vi "Do Set Value.vi"(8 "error in (no error)":errorcluster, 10 "set_value Argument":T3, 11 "Data Cluster in":T1) -> (0 "error out":errorcluster, 3 "Data Cluster out":T1)   [LabVIEW 2025, in "Scripting Server.lvlib"]
uses:
  Scripting Server.lvlib
  Module Data--cluster.ctl
  Config Data.ctl
  set_value Argument--cluster.ctl
  set_value (Reply Payload)--cluster.ctl
  <vilib>/Utility/error.llb/Error Cluster From Error Code.vi
  <vilib>/ErrorRing/Error Ring.xnode
panel:
  out "Class Name":string
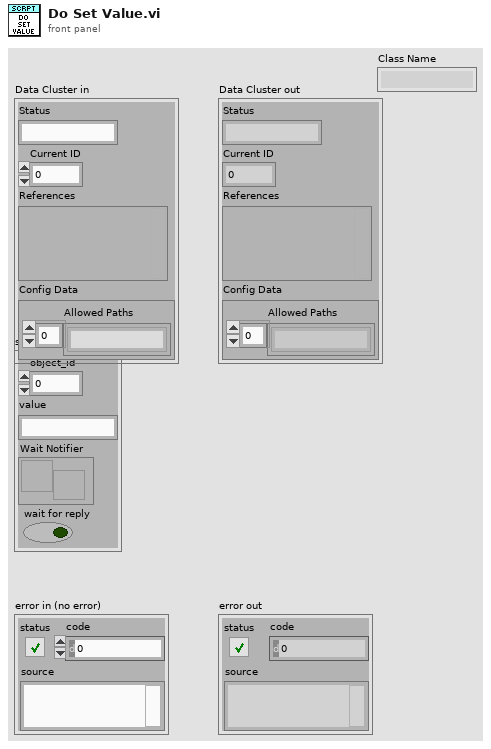
[diagram p1: front panel]
types:
  T1 = typedef "Scripting Server.lvlib/Module Data--cluster.ctl" = cluster{"Status":string, "Current ID":i32, "References":variant, "Config Data":T2}
  T2 = typedef "Scripting Server.lvlib/Config Data.ctl" = cluster{"Allowed Paths":string[]}
  T3 = typedef "Scripting Server.lvlib/set_value Argument--cluster.ctl" = cluster{"object_id":i32, "value":string, "Wait Notifier":refnum<notifier>, "wait for reply":bool}
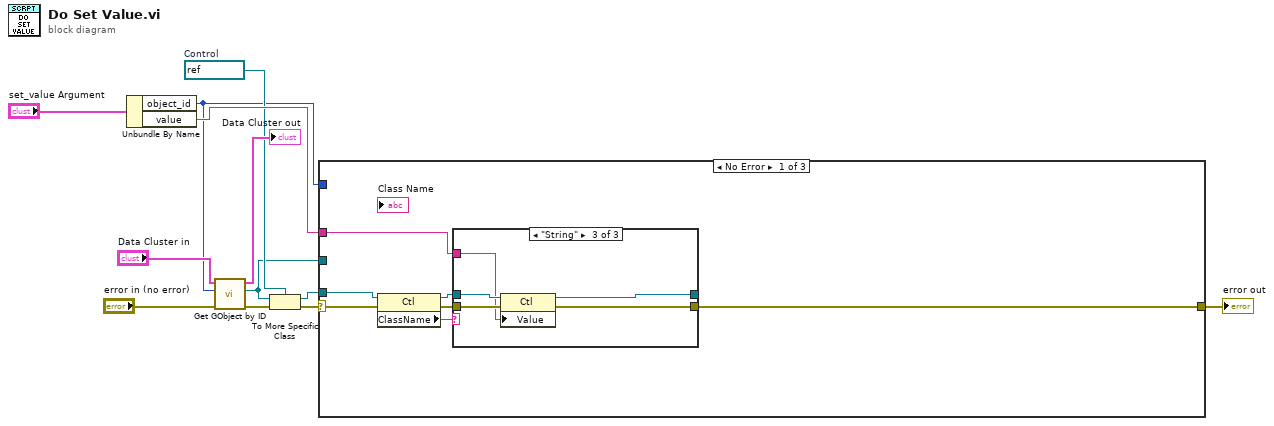
[diagram p0: block diagram]
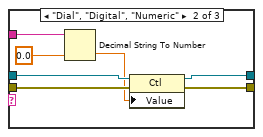
[diagram p3: hidden frame]
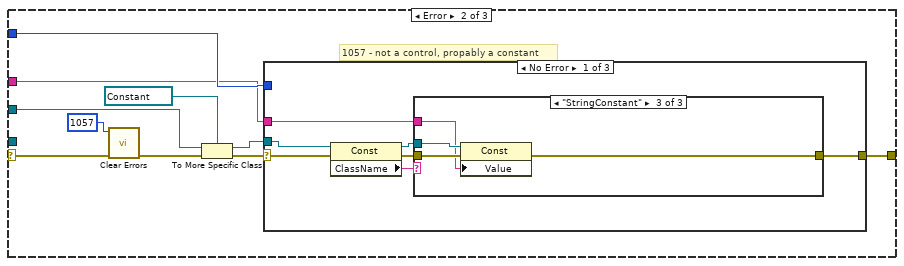
[diagram p4: hidden frame]
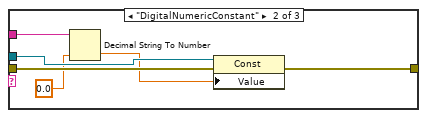
[diagram p6: hidden frame]
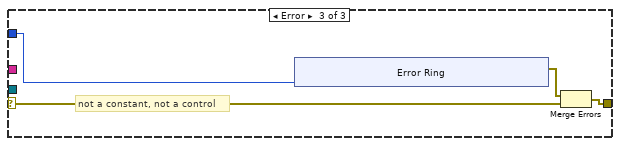
[diagram p8: hidden frame]
diagram:
  w6 = refnum<vi> refnum  # Control
  n1 = Unbundle By Name("set_value Argument") -> ("object_id"=w2:i32, "value"=w7:string)
  n2 = call "Get GObject by ID.vi"("error in (no error)"="error in (no error)", "ID"=w2, "Data Cluster in"="Data Cluster in") -> ("error out"=w4:errorcluster, "gobject"=w1:refnum<vi>, "Data Cluster out"=→"Data Cluster out":T1)  [unwired: 6 in]
  n3 = To More Specific Class(target class=w6, reference=w1, error in=w4) -> (specific class reference=w3:refnum<vi>, error out=w5:errorcluster)
  n4 = case shown="No Error" w5 {
    selector: w5 -> [w19 w43 w74]
    tunnel: w3 -> [w15 _ _]
    tunnel: [w18 w41 w74] -> w8
    tunnel: w7 -> [w17 w37 _]
    tunnel: w2 -> [_ w38 _]
    tunnel: w1 -> [_ w36 _]
    frame No Error {
      n5 = property class="Ctl"(reference=w15, error in=w19) -> (reference out=w14:refnum<vi>, error out=w16:errorcluster, "ClassName"=w13:string)
      n6 = case shown="\"String\"" w13 {
        tunnel: w16 -> [w20 w28 w33]
        tunnel: [w20 w27 w32] -> w18
        tunnel: w14 -> [w21 w26 w31]
        tunnel: [w21 w25 w30] -> _
        tunnel: w17 -> [_ w24 w29]
        frame "False", Default {
        }
        frame "Dial", "Digital", "Numeric" {
          n7 = Decimal String To Number(string=w24, default (0L)=0.0) -> (number=w23:dbl)  [unwired: 1 in, 1 out]
          n8 = property class="Ctl"(reference=w26, error in=w28, "Value"=w23) -> (reference out=w25:refnum<vi>, error out=w27:errorcluster)
        }
        frame "String" {
          n9 = property class="Ctl"(reference=w31, error in=w33, "Value"=w29) -> (reference out=w30:refnum<vi>, error out=w32:errorcluster)
        }
      }
    }
    frame Error {
      # "1057 - not a control, propably a constant"
      n10 = call <vilib>:"Clear Errors.vi"("error in (no error)"=w43, "specific error code to clear (0: all)"=1057) -> ("error out"=w35:errorcluster)  [unwired: 4 in, 1 out]
      n11 = To More Specific Class(target class=refnum<vi> refnum ("reference"), reference=w36, error in=w35) -> (specific class reference=w40:refnum<vi>, error out=w39:errorcluster)
      n12 = case shown="No Error" w39 {
        selector: w39 -> [w48 w62 w66]
        tunnel: [w47 w62 w64] -> w41
        tunnel: w40 -> [w49 _ _]
        tunnel: w38 -> [_ _ w65]
        tunnel: w37 -> [w44 _ _]
        frame No Error {
          n13 = property class="Const"(reference=w49, error in=w48) -> (reference out=w46:refnum<vi>, error out=w50:errorcluster, "ClassName"=w45:string)
          n14 = case shown="\"StringConstant\"" w45 {
            tunnel: w50 -> [w51 w57 w61]
            tunnel: [w51 w56 w60] -> w47
            tunnel: w46 -> [_ w55 w59]
            tunnel: w44 -> [_ w54 w58]
            frame "False", Default {
            }
            frame "DigitalNumericConstant" {
              n15 = Decimal String To Number(string=w54, default (0L)=0.0) -> (number=w53:dbl)  [unwired: 1 in, 1 out]
              n16 = property class="Const"(reference=w55, error in=w57, "Value"=w53) -> (error out=w56:errorcluster)  [unwired: 1 out]
            }
            frame "StringConstant" {
              n17 = property class="Const"(reference=w59, error in=w61, "Value"=w58) -> (error out=w60:errorcluster)  [unwired: 1 out]
            }
          }
        }
        frame Default {
        }
        frame Error {
          # "not a constant, not a control"
          n18 = xnode "Error Ring"("parameter 0"=w65) -> ("error out"=w63:errorcluster)
          n19 = Merge Errors(w63, w66) -> (w64:errorcluster)
        }
      }
    }
    frame Default {
    }
  }
  "error out" <- w8
